vi "Modules - Communications V2.vi"() -> ()   [LabVIEW 2019]
uses:
  Controls/UDP - Event.ctl
  Controls/UDP - Status.ctl
  Controls/Communications - State.ctl
  Controls/eFGV States.ctl
  Controls/Communications - Data Structure.ctl
  Controls/FTDI - Communication.ctl
  Controls/UDP - Command.ctl
  Controls/Communication - Write Data.ctl
  Controls/UDP - Communication.ctl
  Controls/Global - Hold.vi
  Controls/Global - IP Address.vi
  Controls/Global - Handle.vi
  Controls/Global - Comport.vi
  Controls/Global - Device.vi
  Controls/Global - Data UDP.vi
  Controls/Global - Device Type.vi
  Controls/Global - Unit.vi
  Controls/Global - ADC.vi
  Controls/Global - PID.vi
  Controls/Global - System.vi
  Controls/Global - Test.vi
  Controls/Global - Channel.vi
  Controls/Global - Rendezvous.vi
  Controls/FGV States.ctl
panel:
  out "IP Registered":string[](array[string])
  out "Array":cluster{"error out":errorcluster, "IP":string}[](array[cluster])
  out "error out":errorcluster
  in  "timeout ms (25000)":i32=3000
  out "data out":string
  out "Array 2":T3(array[cluster]) {"Data"."Event" items=["Stop", "Running", "PID", "Up Limit", "Down Limit", "Load Limit"]; "Data"."Status" items=["Stop", "Ramp Up", "Ramp Down", "Jog Up", "Jog Down", "PID Mode", "PID Ramp"]}
  out "UDP Conn ref":refnum<k16>
  out "Stop":bool=TRUE
  out "IP":string[](array[string])
  out "Device":string[](array[string])
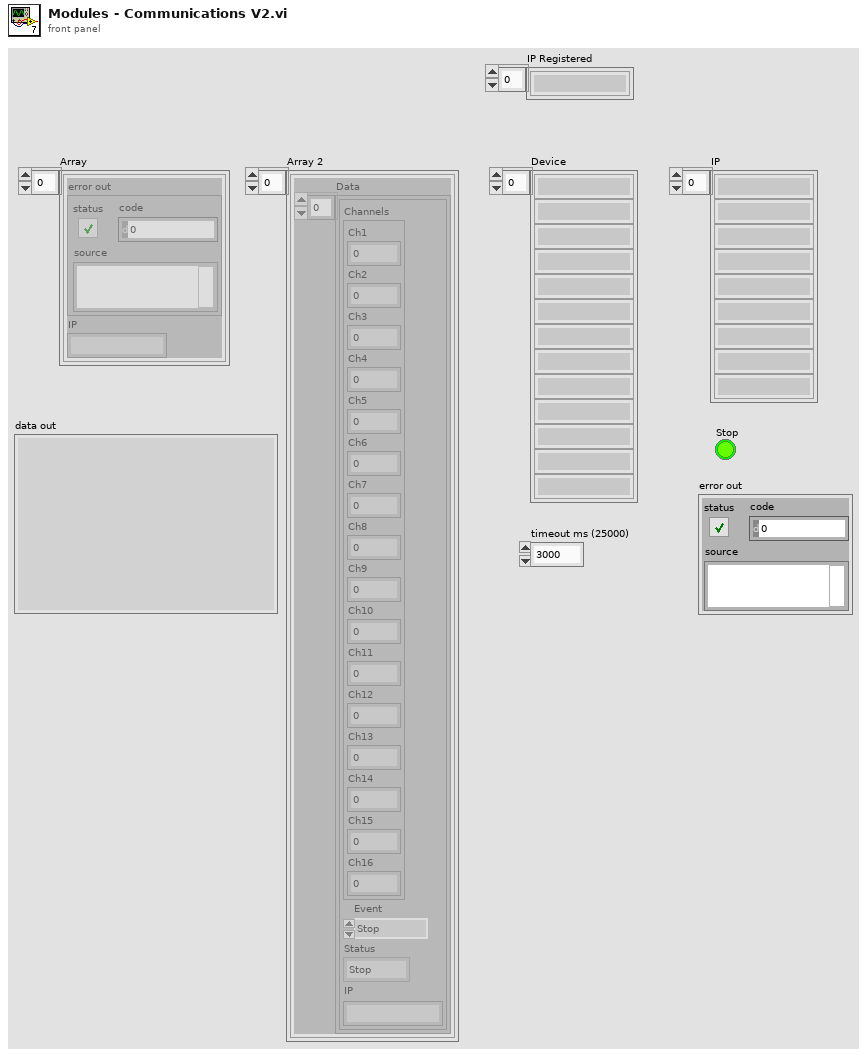
[diagram p1: front panel]
types:
  T1 = typedef "UDP - Event.ctl" = u16
  T2 = typedef "UDP - Status.ctl" = u16
  T3 = cluster{"Data":cluster{"Channels":cluster{"Ch1":sgl, "Ch2":sgl, "Ch3":sgl, "Ch4":sgl, "Ch5":sgl, "Ch6":sgl, "Ch7":sgl, "Ch8":sgl, "Ch9":sgl, "Ch10":sgl, "Ch11":sgl, "Ch12":sgl, "Ch13":sgl, "Ch14":sgl, "Ch15":sgl, "Ch16":sgl}, "Event":T1, "Status":T2, "IP":string}[]}[]
  T4 = cluster{"error out":errorcluster, "name":string}[]
  T5 = typedef "Communications - State.ctl" = enum16{"Init", "Idle", "Command", "Get IP Address", "Release Rendezvous", "Feedback", "Close"}
  T6 = enum32{"Invalid", "Standard", "Closed", "Hidden", "Minimized", "Maximized"}
  T7 = typedef "eFGV States.ctl" = enum16{"Init", "Read", "Write", "Exit"}
  T8 = typedef "Communications - Data Structure.ctl" = cluster{"UDP CMD":T9, "Unit?":bool, "Read Unit":bool[], "Trig?":bool, "UDP Info":cluster{"IP Address":string, "port":string, "UDP ref":refnum<k16>}[], "DataLogger":bool[], "VISA Ref":refnum<event-registration>, "Float":sgl, "Data":T11, "UDP Event Ref":refnum<event-registration>, "UDP ref":refnum<k16>, "Read Sensor":u8}
  T9 = typedef "FTDI - Communication.ctl" = cluster{"IP":string, "CMD":T10, "Port":string, "Datalog?":bool, "Float":dbl}
  T10 = typedef "UDP - Command.ctl" = enum16{"Stop", "Jog Up", "Jog Down", "Ramp Up", "Ramp Down", "PID Target", "PID Ramp", "Disp Run", "Read Ch Data", "Zero Channel", "Zero Disp", "Read Sensor", "Write Sensor", "Read ADC", "Write ADC", "Read PID", "Write PID", "Read Test", "Write Test", "Read System", "Write System", "Read Datalog", "Read Datalog Sensor"}
  T11 = typedef "Communication - Write Data.ctl" = cluster{"Test":cluster{"Target Load":sgl, "Target Disp":sgl, "Rate":sgl, "Speed":sgl}, "Sensor":cluster{"Name":string[], "Unit":string[], "Decimal Point":u8[], "Ch Log":u8[], "H Alarm":u8[], "L Alarm":u8[], "H Limit":sgl[], "L Limit":sgl[], "Filter":u8[], "Gain":u8[], "Calib Type":u32[]}, "PID":cluster{"SP":sgl, "PV":sgl, "kP":sgl, "kI":sgl, "kD":sgl, "FF":sgl, "Err Band":sgl, "Max":i32, "Min":i32, "Ts":u32, "Out":i32, "Mode":u8}, "ADC":cluster{"Active Ch":u8[], "Filter Type":u8, "Post Filter":u8[], "Gain":u8[], "FS":u16, "IntOC":u8, "IntFC":u8, "SysOC":u8, "Cofficient":dbl[], "K":dbl[], "Max":i32}, "System":cluster{"Out Type":u8, "Inverse":u8, "Monitor":u8, "Reserve":u8, "ACC Time":u32, "Pulse Rev":u32, "Stroke":u32, "Auto Off":u32, "Gear Ratio":sgl, "Pitch":sgl, "Max Speed":u32, "Jog Speed":u32, "Disp Coff":sgl, "Max Load":u32}, "Index":enum16{"Ch1", "Ch2", "Ch3", "Ch4", "Ch5", "Ch6", "Ch7", "Ch8", "Ch9", "Ch10", "Ch11", "Ch12", "Ch13", "Ch14", "Ch15", "Ch16"}, "Datalog":enum16{"Ch1-Ch16", "Ch17-Ch32", "Ch32-Ch48", "Ch49-Ch64", "Empty"}}
  T12 = cluster{"IP Address":string, "port":string, "UDP ref":refnum<k16>}
  T13 = enum16{"Ch1-Ch16", "Ch17-Ch32", "Ch32-Ch48", "Ch49-Ch64", "Empty"}
  T14 = cluster{"IP Address":string, "port":string, "UDP ref":refnum<k16>}[]
  T15 = typedef "FGV States.ctl" = enum16{"Read", "Write"}
  T16 = cluster{"Target Load":sgl, "Target Disp":sgl, "Rate":sgl, "Ch4":sgl}
  T17 = cluster{"Name":string[], "Unit":string[], "Decimal Point":u8[], "Ch Log":u8[], "H Alarm":u8[], "L Alarm":u8[], "H Limit":sgl[], "L Limit":sgl[], "Filter":u8[], "Gain":u8[], "Calib Type":u32[]}
  T18 = cluster{"SP":sgl, "PV":sgl, "kP":sgl, "kI":sgl, "kD":sgl, "FF":sgl, "Err Band":sgl, "Max":i32, "Min":i32, "Ts":u32, "Out":i32, "Mode":u8}
  T19 = cluster{"Active Ch":u8[], "Filter Type":u8, "Post Filter":u8[], "Gain":u8[], "FS":u16, "IntOC":u8, "IntFC":u8, "SysOC":u8, "Cofficient":dbl[], "K":dbl[], "Max":i32}
  T20 = cluster{"Out Type":u8, "Inverse":u8, "Monitor":u8, "Reserve":u8, "ACC Time":u32, "Pulse Rev":u32, "Stroke":u32, "Auto Off":u32, "Gear Ratio":sgl, "Pitch":sgl, "Max Speed":u32, "Jog Speed":u32, "Disp Coff":sgl, "Max Load":u32}
  T21 = cluster{"Name":string[], "Unit":string[], "Decimal Point":u8[], "Ch Log":u8[], "H Alarm":u8[], "L Alarm":u8[], "H Limit":sgl[], "L Limit":sgl[], "Filter":u8[], "Gain":u8[], "Calib Type":u32[]}[]
  T22 = cluster{"Active Ch":u8[], "Filter Type":u8, "Post Filter":u8[], "Gain":u8[], "FS":u16, "IntOC":u8, "IntFC":u8, "SysOC":u8, "Cofficient":dbl[], "K":dbl[], "Max":i32}[]
  T23 = cluster{"SP":sgl, "PV":sgl, "kP":sgl, "kI":sgl, "kD":sgl, "FF":sgl, "Err Band":sgl, "Max":i32, "Min":i32, "Ts":u32, "Out":i32, "Mode":u8}[]
  T24 = cluster{"Out Type":u8, "Inverse":u8, "Monitor":u8, "Reserve":u8, "ACC Time":u32, "Pulse Rev":u32, "Stroke":u32, "Auto Off":u32, "Gear Ratio":sgl, "Pitch":sgl, "Max Speed":u32, "Jog Speed":u32, "Disp Coff":sgl, "Max Load":u32}[]
  T25 = cluster{"Target Load":sgl, "Target Disp":sgl, "Rate":sgl, "Speed":sgl}
  T26 = cluster{"Target Load":sgl, "Target Disp":sgl, "Rate":sgl, "Speed":sgl}[]
  T27 = cluster{"Channels":cluster{"Ch1":sgl, "Ch2":sgl, "Ch3":sgl, "Ch4":sgl, "Ch5":sgl, "Ch6":sgl, "Ch7":sgl, "Ch8":sgl, "Ch9":sgl, "Ch10":sgl, "Ch11":sgl, "Ch12":sgl, "Ch13":sgl, "Ch14":sgl, "Ch15":sgl, "Ch16":sgl}, "Event":T1, "Status":T2, "IP":string}[]
  T28 = cluster{"Data":cluster{"Channels":cluster{"Ch1":sgl, "Ch2":sgl, "Ch3":sgl, "Ch4":sgl, "Ch5":sgl, "Ch6":sgl, "Ch7":sgl, "Ch8":sgl, "Ch9":sgl, "Ch10":sgl, "Ch11":sgl, "Ch12":sgl, "Ch13":sgl, "Ch14":sgl, "Ch15":sgl, "Ch16":sgl}, "Event":T1, "Status":T2, "IP":string}[]}
  T29 = typedef "Rendezvous RefNum" = refnum<k1>
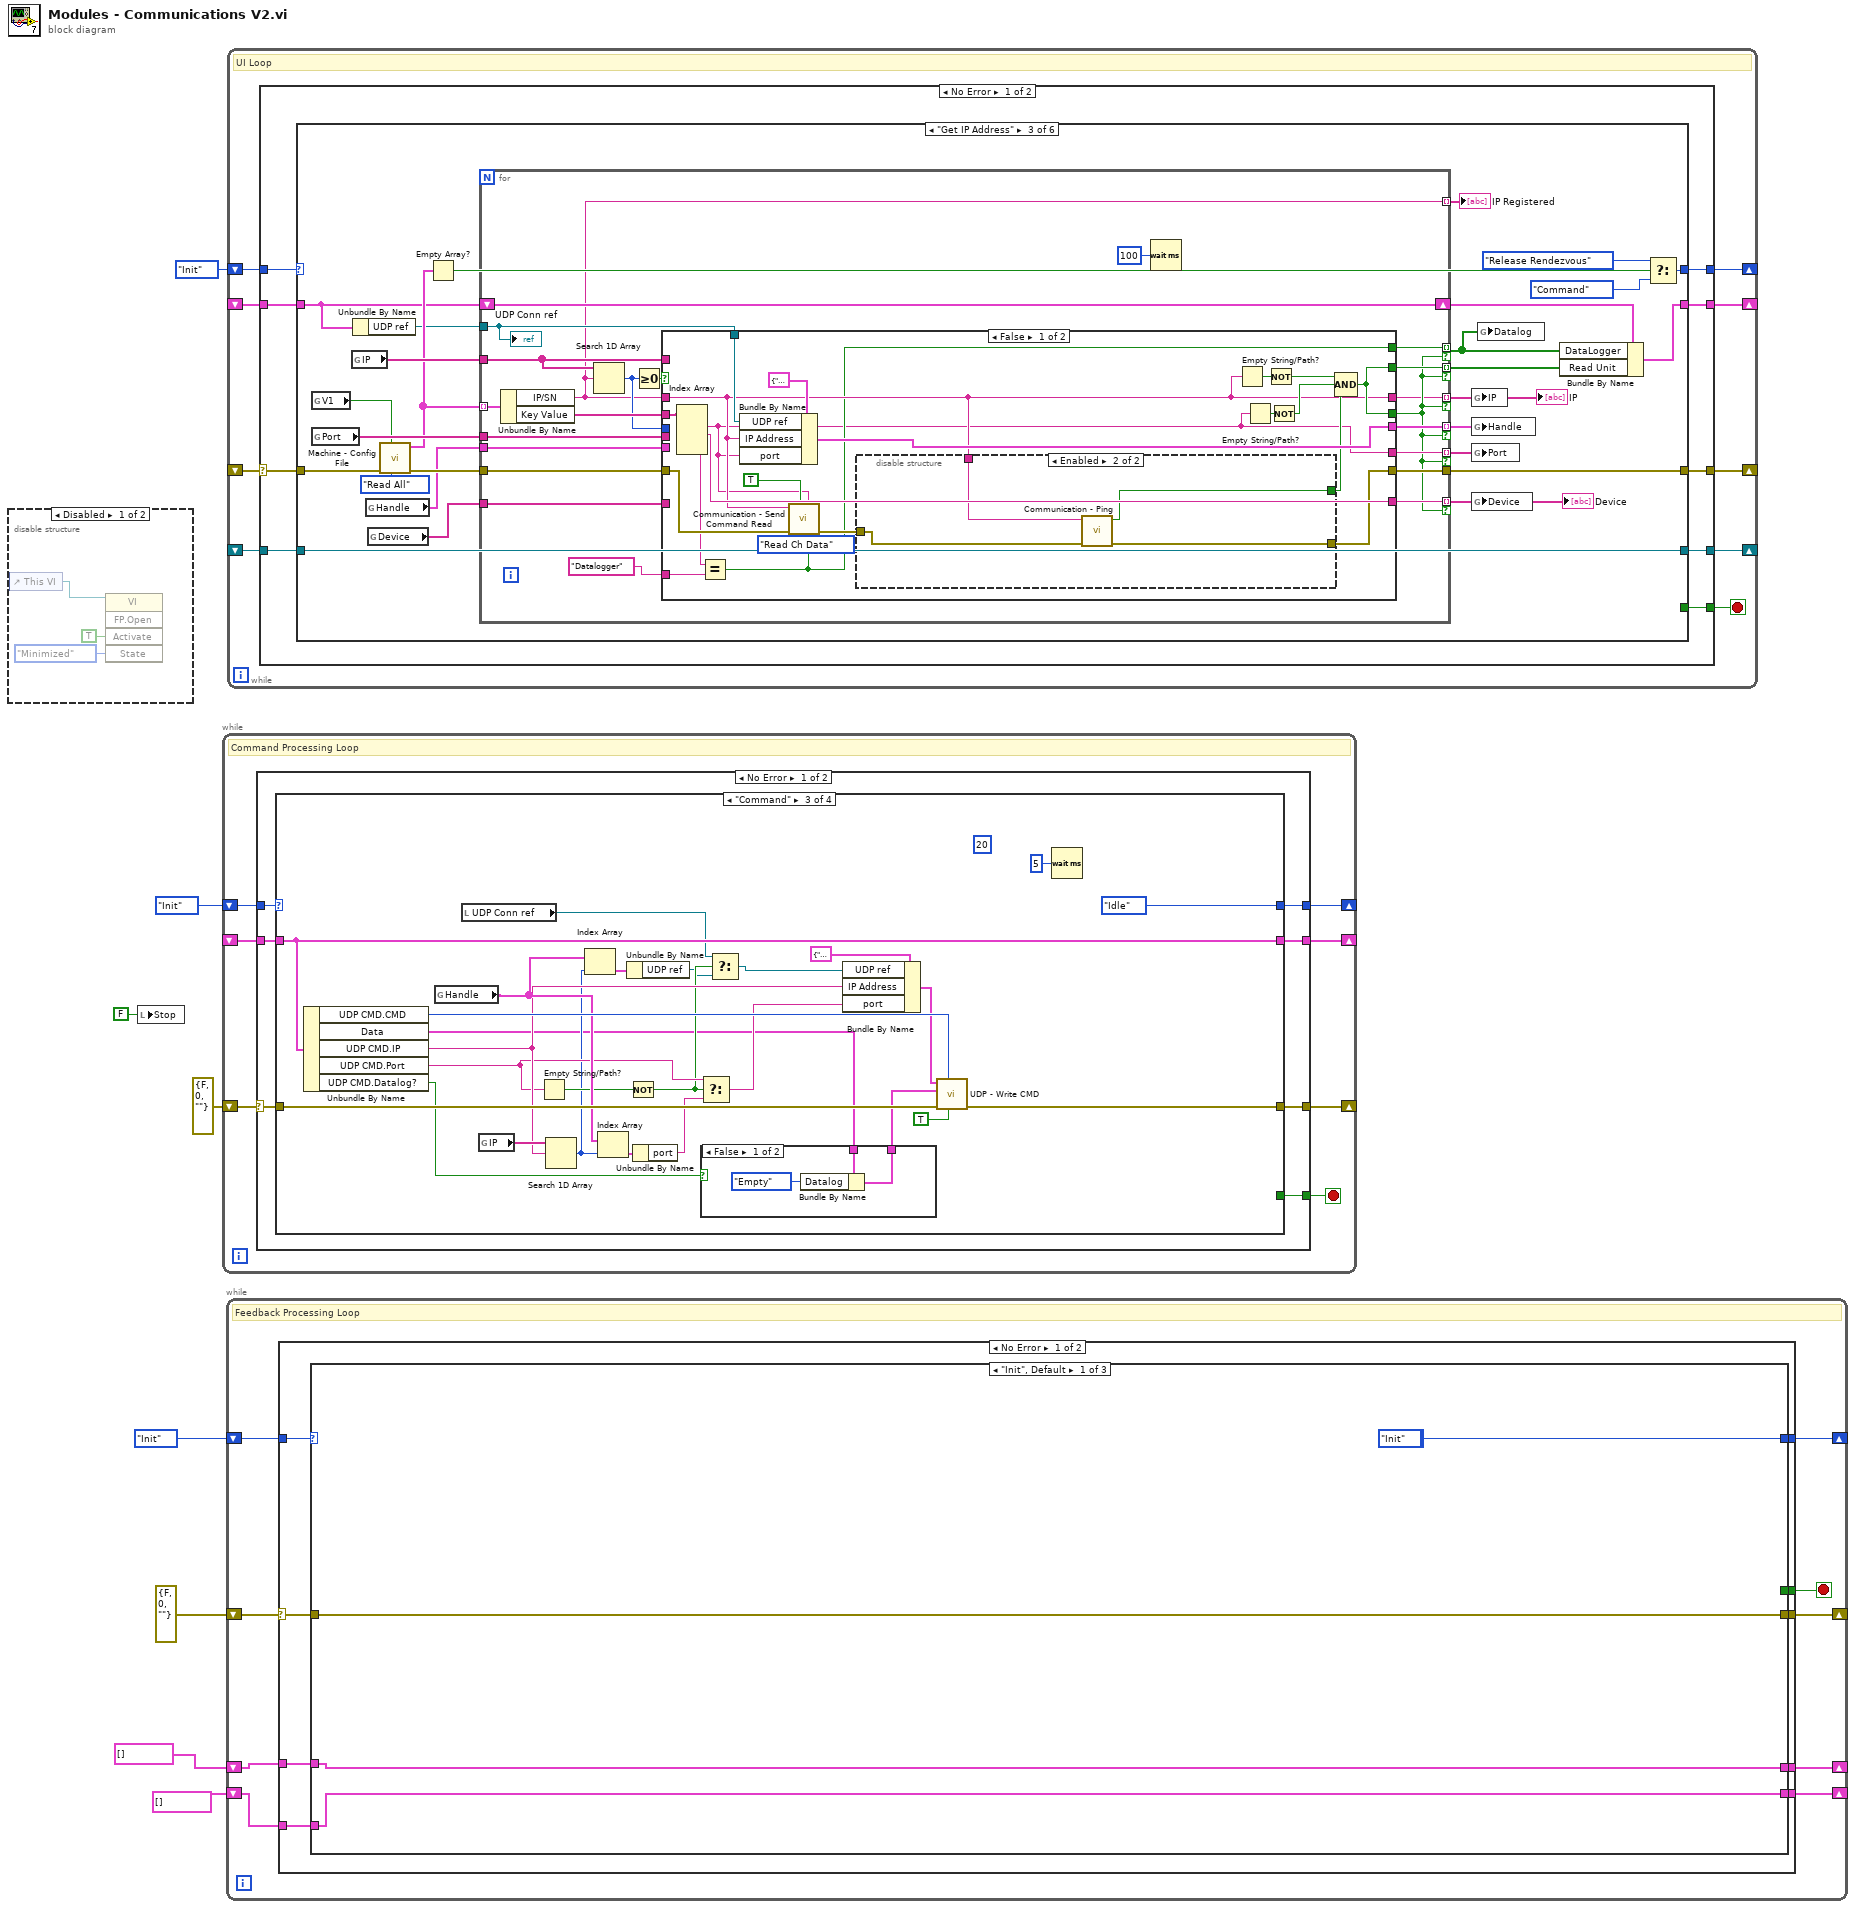
[diagram p0: block diagram]
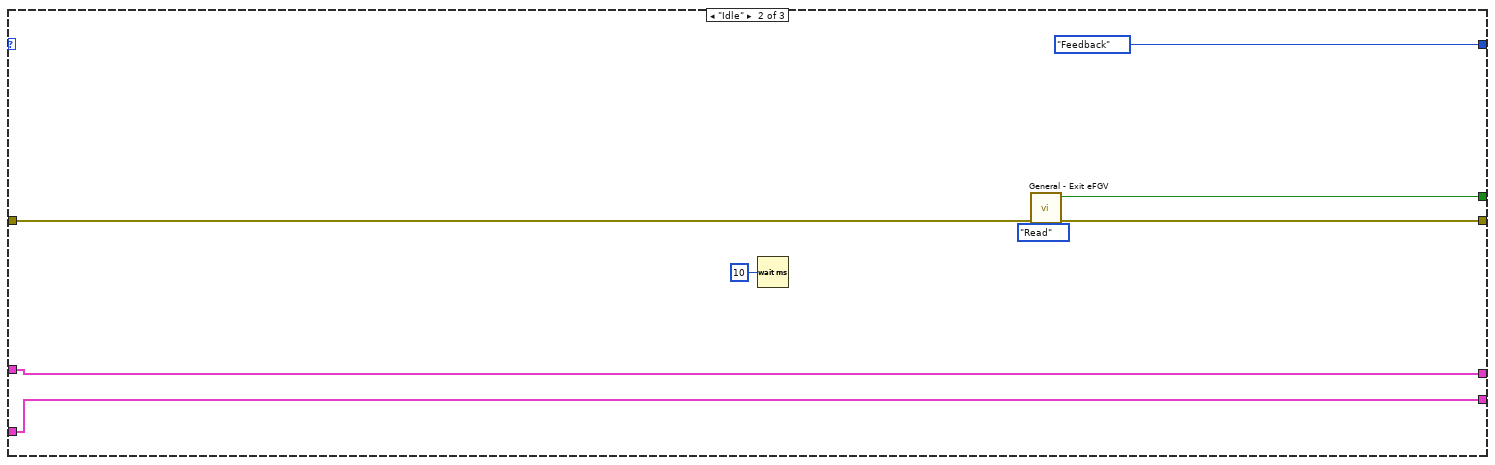
[diagram p3: hidden frame]
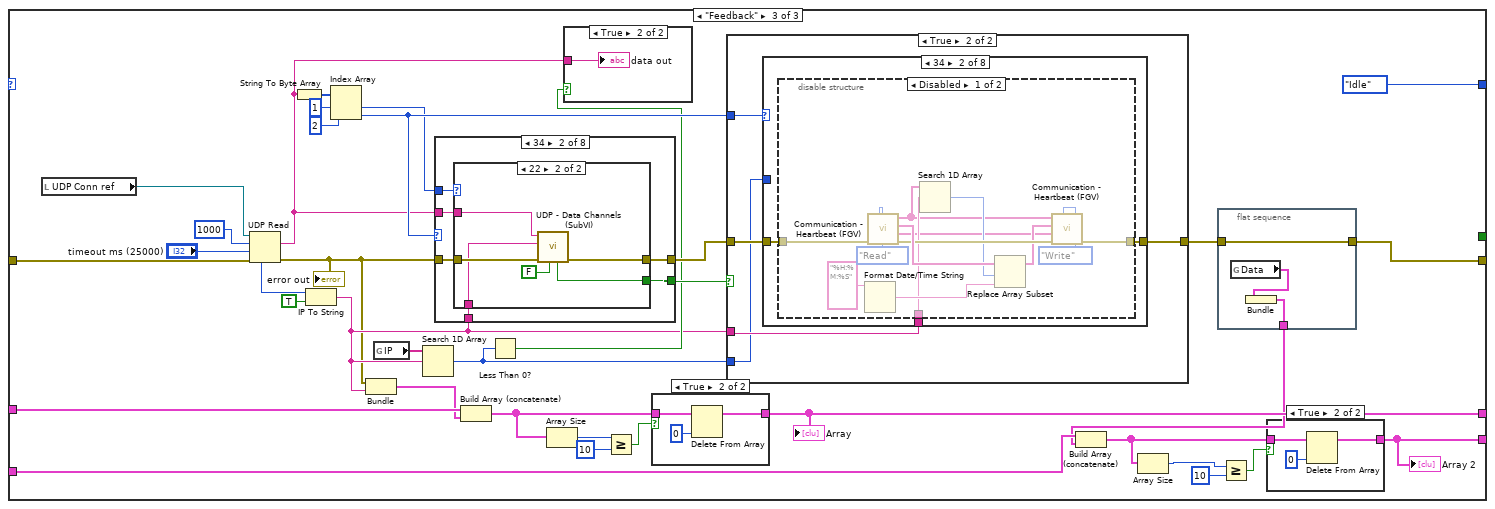
[diagram p4: hidden frame]
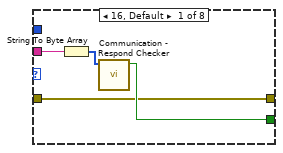
[diagram p8: hidden frame]
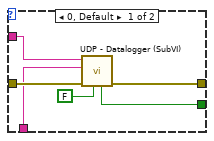
[diagram p9: hidden frame]
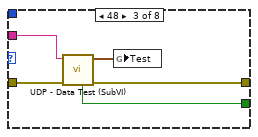
[diagram p10: hidden frame]
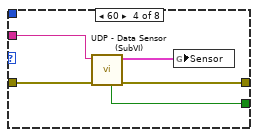
[diagram p11: hidden frame]
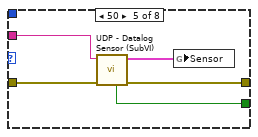
[diagram p12: hidden frame]
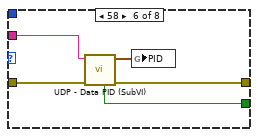
[diagram p13: hidden frame]
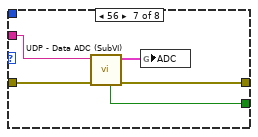
[diagram p14: hidden frame]
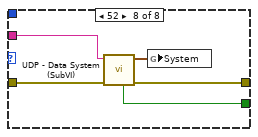
[diagram p15: hidden frame]
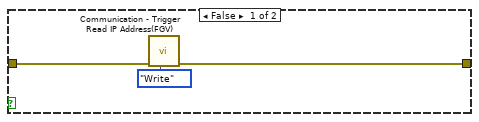
[diagram p16: hidden frame]
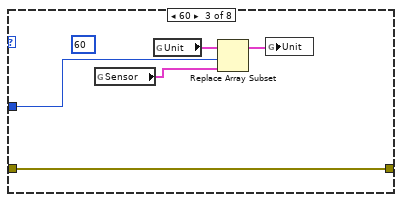
[diagram p19: hidden frame]
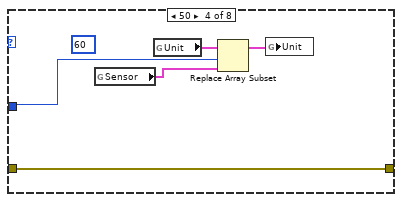
[diagram p20: hidden frame]
diagram:
  (unwired) Communications_-_State."Init"
  (unwired) Communications_-_State."Init"
  n1 = disable-structure shown="Disabled" {
    frame Disabled {
      n2 = control-ref of="This VI"() -> (w11:refnum<vi>)
      n3 = invoke class="VI" method="FP.Open"(reference=w11, "Activate"=TRUE ("Activate?"), "State"=T6."Minimized") -> ()  [unwired: 2 in, 5 out]
    }
    frame Enabled {
    }
  }
  n4 = local write "Stop"(FALSE ("Stop")) -> ()
  n5 = while {
    shift-right: [w17] -> _
    shift-left: errorcluster {"status"=FALSE, "code"=0, "source"=""} ("error IO") -> [w18]
    shift-right: [w15] -> _
    shift-left: Communications_-_State."Init" -> [w16]
    shift-right: [w13] -> _
    shift-left: _ -> [w12]
    stop <- w14 stop-if-true
    # "Command Processing Loop"
    n6 = case shown="No Error" w18 {
      selector: w18 -> [w24 w108]
      tunnel: [w25 w101] -> w17
      tunnel: w16 -> [w23 _]
      tunnel: [w22 Communications_-_State."Idle"] -> w15
      tunnel: [w21 _] -> w14
      tunnel: [w20 w110] -> w13
      tunnel: w12 -> [w19 w110]
      frame No Error {
        n7 = case shown="\"Command\"" w23 {
          tunnel: [w29 w43 w77 w98] -> w25
          tunnel: w24 -> [w27 w42 w87 w98]
          tunnel: [Communications_-_State."Idle" w37 Communications_-_State."Idle" Communications_-_State."Close"] -> w22
          tunnel: [_ _ _ TRUE] -> w21
          tunnel: [w31 w41 w86 w95] -> w20
          tunnel: w19 -> [_ w40 w86 w95]
          frame "Init", Default {
            n8 = call "Communication - UDP Command (eFGV).vi"("Action"=eFGV_States."Read", "error in"=w27) -> ("error out"=w30:errorcluster, "UDP Ref"=w28:refnum<user-event>)  [unwired: 7 in, 1 out]
            n9 = register-events(error in=w30, w28) -> (reference out=w26:refnum<event-registration>, error out=w29:errorcluster)  [unwired: 1 in]
            n10 = Bundle By Name(cluster=T8 {"UDP CMD"={"IP"="", "CMD"=enum."Stop", "Port"="", "Datalog?"=FALSE, "Float"=0.0}, "Unit?"=FALSE, "Read Unit"=[], "Trig?"=FALSE, "UDP Info"=[], "DataLogger"=[], "VISA Ref"=refnum, "Float"=0.0, "Data"={"Test"={"Target Load"=0.0, "Target Disp"=0.0, "Rate"=0.0, "Speed"=0.0}, "Sensor"={"Name"=[], "Unit"=[], "Decimal Point"=[], "Ch Log"=[], "H Alarm"=[], "L Alarm"=[], "H Limit"=[], "L Limit"=[], "Filter"=[], "Gain"=[], "Calib Type"=[]}, "PID"={"SP"=-2.7823365e-08, "PV"=-3.023652e-13, "kP"=8.5432666e-24, "kI"=2.29252e-41, "kD"=1.570387e-38, "FF"=25.0, "Err Band"=0.0, "Max"=15, "Min"=-7, "Ts"=1886611780, "Out"=0, "Mode"=0}, "ADC"={"Active Ch"=[255, 255, 255, 0, 0, 0, 0, 0], "Filter Type"=2, "Post Filter"=[1, 1, 1, 1, 0, 200, 66, 184], "Gain"=[0, 0, 0, 0, 0, 122, 68, 0], "FS"=32, "IntOC"=0, "IntFC"=255, "SysOC"=255, "Cofficient"=[1.0, 1.0, 1.0, 1.0, 1.0, 1.0, 1.0, 1.0], "K"=[1.2450000047683716, 1.2450000047683716], "Max"=1048576}, "System"={"Out Type"=0, "Inverse"=0, "Monitor"=0, "Reserve"=0, "ACC Time"=0, "Pulse Rev"=0, "Stroke"=0, "Auto Off"=0, "Gear Ratio"=0.0, "Pitch"=0.0, "Max Speed"=0, "Jog Speed"=0, "Disp Coff"=0.0, "Max Load"=0}, "Index"=enum."Ch1", "Datalog"=enum."Empty"}, "UDP Event Ref"=refnum, "UDP ref"=refnum, "Read Sensor"=0}, "UDP Event Ref"=w26) -> (w31:T8)
          }
          frame "Idle" {
            n11 = Unbundle By Name(w40) -> ("UDP Event Ref"=w44:refnum<event-registration>)
            n12 = event shown="[1] <UDP Ref>: User Event" {
              selector: w44 -> [_ _]
              dyn-events: _ -> [_ _]
              timeout: 1000 -> [_ _]
              tunnel: [w50 Communications_-_State."Command" ("f")] -> w38
              tunnel: [w47 w54] -> w43
              tunnel: w42 -> [w47 w54]
              tunnel: [w45 w62] -> w41
              tunnel: w40 -> [w45 w61]
              event Timeout {
                n13 = event-data() -> ()  [unwired: 1 in, 1 out]
                n14 = local read "Stop"() -> (w49:bool)
                n15 = Select(t=Communications_-_State."Close", s=w49, f=Communications_-_State."Idle") -> (s? t:f=w50:T5)
              }
              event User Event {
                n16 = event-data() -> ("IP"=w56:string, "CMD"=w60:T10, "Data"=w51:T11, "Port"=w53:string, "Datalog?"=w52:bool)  [unwired: 1 in]
                n17 = global read "Global - IP Address.vi" "IP"() -> (w59:string[])
                n18 = Index Array(array=w59, index=0) -> (element=w57:string)
                n19 = Equal?(x=w57, y=w56) -> ()  [unwired: 1 out]
                n20 = Bundle By Name(cluster=w61, "UDP CMD.IP"=w56, "UDP CMD.CMD"=w60, "Data"=w51, "UDP CMD.Port"=w53, "UDP CMD.Datalog?"=w52) -> (w62:T8)
              }
            }
            n21 = global read "Global - Hold.vi" "Hold"() -> (w39:bool)
            n22 = Select(t=Communications_-_State."Idle", s=w39, f=w38) -> (s? t:f=w37:T5)
          }
          frame "Command" {
            (unwired) 20
            n23 = Unbundle By Name(w86) -> ("UDP CMD.CMD"=w85:T10, "Data"=w65:T11, "UDP CMD.IP"=w79:string, "UDP CMD.Port"=w73:string, "UDP CMD.Datalog?"=w64:bool)
            n24 = global read "Global - Handle.vi" "Handle"() -> (w81:T14)
            n25 = local read "UDP Conn ref"() -> (w68:refnum<k16>)
            n26 = global read "Global - IP Address.vi" "IP"() -> (w83:string[])
            n27 = Empty String/Path?(string/path=w73) -> (empty?=w74:bool)
            n28 = Search 1D Array(1D array=w83, element=w79) -> (index of element=w67:i32)  [unwired: 1 in]
            n29 = Index Array(array=w81, index=w67) -> (element=w80:T12)
            n30 = Index Array(array=w81, index=w67) -> (element=w78:T12)
            n31 = Unbundle By Name(w80) -> ("UDP ref"=w69:refnum<k16>)
            n32 = Not(x=w74) -> (.not. x?=w70:bool)
            n33 = Unbundle By Name(w78) -> ("port"=w72:string)
            n34 = Select(t=w73, s=w70, f=w72) -> (s? t:f=w71:string)
            n35 = case shown="False" w64 {
              tunnel: w65 -> [w91 w94]
              tunnel: [w90 w93] -> w63
              frame False {
                n36 = Bundle By Name(cluster=w91, "Datalog"=T13."Empty") -> (w90:T11)
              }
              frame True {
                n37 = Bundle By Name(cluster=w94, "Datalog"=T13."Ch1-Ch16") -> (w93:T11)
              }
            }
            n38 = Select(t=w68, s=w70, f=w69) -> (s? t:f=w66:refnum<k16>)
            n39 = Bundle By Name(cluster=T12 {"IP Address"="", "port"="", "UDP ref"=refnum} ("element"), "UDP ref"=w66, "IP Address"=w79, "port"=w71) -> (w76:T12)
            n40 = call "UDP - Write CMD.vi"("V2"=TRUE, "CMD"=w85, "error in"=w87, "Data"=w63, "UDP Info"=w76) -> ("error out"=w77:errorcluster)  [unwired: 6 out]
            n41 = Wait (ms)(milliseconds to wait=u32 5) -> ()  [unwired: 1 out]
          }
          frame "Close" {
          }
        }
      }
      frame Error {
        n42 = global read "Global - IP Address.vi" "IP"() -> (w107:string[])
        n43 = Unbundle By Name(w108) -> ("source"=w103:string)
        n44 = Index Array(array=w107, index=0) -> (element=w105:string)
        n45 = Concatenate Strings(w105, " - " ("string"), w103) -> (w99:string)
        n46 = call <vilib>:"Clear Errors.vi"("error in (no error)"=w108) -> ("error out"=w102:errorcluster)  [unwired: 5 in, 1 out]
        n47 = call "General - Error Log eFGV.vi"("eFGV States"=eFGV_States."Write", "error in (no error)"=w102, "Error In"=w99) -> ("error out"=w101:errorcluster)  [unwired: 6 in, 2 out]
        n48 = Wait (ms)(milliseconds to wait=u32 100) -> ()  [unwired: 1 out]
      }
    }
  }
  n49 = while {
    shift-right: [w118] -> _
    shift-left: Communications_-_State."Init" -> [w119]
    shift-right: [w117] -> _
    shift-left: errorcluster {"status"=FALSE, "code"=0, "source"=""} ("error IO") -> [w120]
    shift-right: [w115] -> _
    shift-left: T4 [] -> [w114]
    shift-right: [w113] -> _
    shift-left: T3 [] -> [w112]
    stop <- w116 stop-if-true
    # "Feedback Processing Loop"
    n50 = case shown="No Error" w120 {
      selector: w120 -> [w126 w303]
      tunnel: w119 -> [w129 _]
      tunnel: [w128 Communications_-_State."Idle"] -> w118
      tunnel: [w127 w300] -> w117
      tunnel: [w125 _] -> w116
      tunnel: [w124 w299] -> w115
      tunnel: w114 -> [w123 w299]
      tunnel: [w122 w298] -> w113
      tunnel: w112 -> [w121 w298]
      frame No Error {
        n51 = case shown="\"Init\", Default" w129 {
          tunnel: [Communications_-_State."Idle" Communications_-_State."Feedback" Communications_-_State."Idle"] -> w128
          tunnel: [w132 w139 w150] -> w127
          tunnel: w126 -> [w132 w138 w165]
          tunnel: [_ w137 _] -> w125
          tunnel: [w131 w135 w158] -> w124
          tunnel: w123 -> [w131 w135 w162]
          tunnel: [w130 w134 w145] -> w122
          tunnel: w121 -> [w130 w134 w153]
          frame "Init", Default {
            (unwired) Communications_-_State."Init"
          }
          frame "Idle" {
            n52 = Wait (ms)(milliseconds to wait=u32 10) -> ()  [unwired: 1 out]
            n53 = call "General - Exit eFGV.vi"("eFGV States"=eFGV_States."Read", "error in (no error)"=w138) -> ("error out"=w139:errorcluster, "Exit Out"=w137:bool)  [unwired: 7 in, 1 out]
          }
          frame "Feedback" {
            n54 = local read "UDP Conn ref"() -> (w164:refnum<k16>)
            n55 = UDP Read(connection ID=w164, max size (548)=1000, timeout ms (25000)="timeout ms (25000)", 8:w165) -> (data out=w163:string, error out=w143:errorcluster, 6:w170:u32)  [unwired: 2 out]
            "error out" <- w143
            n56 = String To Byte Array(string=w163) -> (unsigned byte array=w174:u8[])
            n57 = IP To String(1:TRUE ("dot notation? (F)"), 2:w170) -> (0:w144:string)
            n58 = Index Array(array=w174, index #1=1 ("index"), index #2=2 ("index")) -> (element #1=w175:u8, element #2=w176:u8)
            n59 = Bundle("error out"=w143, "name"=w144) -> (w142:cluster{"error out":errorcluster, "name":string})  [unwired: 1 in]
            n60 = global read "Global - IP Address.vi" "IP"() -> (w173:string[])
            n61 = Search 1D Array(1D array=w173, element=w144) -> (index of element=w148:i32)  [unwired: 1 in]
            n62 = case shown="34" w176 {
              tunnel: [w191 w199 w216 w221 w226 w231 w236 w241] -> w172
              tunnel: [w192 w198 w215 w220 w225 w230 w235 w240] -> w171
              tunnel: w143 -> [w191 w195 w213 w218 w223 w228 w233 w238]
              tunnel: w163 -> [w190 w197 w212 w217 w222 w227 w232 w237]
              tunnel: w175 -> [_ w196 _ _ _ _ _ _]
              tunnel: w144 -> [_ w194 _ _ _ _ _ _]
              frame 16, Default {
                n63 = String To Byte Array(string=w190) -> (unsigned byte array=w193:u8[])
                n64 = call "Communication - Respond Checker.vi"("Read Data"=w193) -> ("Success"=w192:bool)  [unwired: 10 in]
              }
              frame 34 {
                n65 = case shown="22" w196 {
                  tunnel: [w203 w211] -> w199
                  tunnel: [w202 w210] -> w198
                  tunnel: w197 -> [w201 w208]
                  tunnel: w195 -> [w204 w207]
                  tunnel: w194 -> [w200 w206]
                  frame 0, Default {
                    n66 = call "UDP - Datalogger (SubVI).vi"("test?"=FALSE, "error in"=w204, "IP"=w200, "data in"=w201) -> ("error out"=w203:errorcluster, "Success"=w202:bool)  [unwired: 5 in, 1 out]
                  }
                  frame 22 {
                    n67 = call "UDP - Data Channels (SubVI).vi"("test?"=FALSE, "error in"=w207, "IP"=w206, "data in"=w208) -> ("error out"=w211:errorcluster, "Success"=w210:bool)  [unwired: 2 in, 4 out]
                  }
                }
              }
              frame 48 {
                n68 = call "UDP - Data Test (SubVI).vi"("error in"=w213, "data in"=w212) -> ("error out"=w216:errorcluster, "Data Test"=w214:T16, "Success"=w215:bool)  [unwired: 7 in]
                n69 = global write "Global - Data UDP.vi" "Test"(w214) -> ()
              }
              frame 60 {
                n70 = call "UDP - Data Sensor (SubVI).vi"("error in"=w218, "String"=w217) -> ("error out"=w221:errorcluster, "Sensor Out"=w219:T17, "Success"=w220:bool)  [unwired: 7 in]
                n71 = global write "Global - Data UDP.vi" "Sensor"(w219) -> ()
              }
              frame 50 {
                n72 = call "UDP - Datalog Sensor (SubVI).vi"("error in"=w223, "String"=w222) -> ("error out"=w226:errorcluster, "Sensor Out"=w224:T17, "Success"=w225:bool)  [unwired: 7 in]
                n73 = global write "Global - Data UDP.vi" "Sensor"(w224) -> ()
              }
              frame 58 {
                n74 = call "UDP - Data PID (SubVI).vi"("error in (no error)"=w228, "Data"=w227) -> ("error out"=w231:errorcluster, "PID Setting"=w229:T18, "Success"=w230:bool)  [unwired: 7 in]
                n75 = global write "Global - Data UDP.vi" "PID"(w229) -> ()
              }
              frame 56 {
                n76 = call "UDP - Data ADC (SubVI).vi"("error in (no error)"=w233, "Data"=w232) -> ("error out"=w236:errorcluster, "Data ADC"=w234:T19, "Success"=w235:bool)  [unwired: 7 in]
                n77 = global write "Global - Data UDP.vi" "ADC"(w234) -> ()
              }
              frame 52 {
                n78 = call "UDP - Data System (SubVI).vi"("error in (no error)"=w238, "Data"=w237) -> ("error out"=w241:errorcluster, "Data System"=w239:T20, "Success"=w240:bool)  [unwired: 7 in]
                n79 = global write "Global - Data UDP.vi" "System"(w239) -> ()
              }
            }
            n80 = Build Array (concatenate)(w162, w142) -> (w159:T4)
            n81 = Less Than 0?(x=w148) -> (x < 0?=w147:bool)
            n82 = Array Size(array=w159) -> (size(s)=w161:i32)
            n83 = case shown="True" w147 {
              tunnel: w163 -> [_ w178]
              frame False {
              }
              frame True {
                "data out" <- w178
              }
            }
            n84 = Greater Or Equal?(x=w161, y=10) -> (x >= y?=w157:bool)
            n85 = case shown="True" w157 {
              tunnel: w159 -> [w186 w189]
              tunnel: [w186 w188] -> w158
              frame False {
              }
              frame True {
                n86 = Delete From Array(array=w189, index=0) -> (array with subset deleted=w188:T4)  [unwired: 1 in, 1 out]
              }
            }
            "Array" <- w158
            n87 = case shown="True" w171 {
              tunnel: w172 -> [w242 w248]
              tunnel: [w243 w247] -> w149
              tunnel: w176 -> [_ w249]
              tunnel: w148 -> [_ w245]
              tunnel: w144 -> [_ w246]
              frame False {
                n88 = call "Communication - Trigger Read IP Address(FGV).vi"("Action"=eFGV_States."Write", "error in"=w242) -> ("error out"=w243:errorcluster)  [unwired: 7 in, 2 out]
              }
              frame True {
                n89 = case shown="34" w249 {
                  tunnel: w248 -> [w250 w253 w269 w274 w279 w287 w292 w297]
                  tunnel: [w250 w252 w269 w274 w279 w287 w292 w297] -> w247
                  tunnel: w245 -> [_ _ w268 w273 w278 w283 w288 w293]
                  tunnel: w246 -> [_ w251 _ _ _ _ _ _]
                  frame 0, Default {
                  }
                  frame 34 {
                    n90 = disable-structure shown="Disabled" {
                      disable-tunnel: w253 -> [w259 w267]
                      disable-tunnel: [w258 w267] -> w252
                      disable-tunnel: w251 -> [w257 _]
                      frame Disabled {
                        n91 = Format Date/Time String(time format string (%c)="%H:%M:%S") -> (date/time string=w263:string)  [unwired: 2 in]
                        n92 = call "Communication - Heartbeat (FGV).vi"("Action"=FGV_States."Read", "error in (no error)"=w259) -> ("error out"=w265:errorcluster, "Previous Out"=w254:string[], "Timestamp Out"=w266:string[], "IP Out"=w255:string[])  [unwired: 6 in]
                        n93 = Search 1D Array(1D array=w255, element=w257) -> (index of element=w256:i32)  [unwired: 1 in]
                        n94 = Replace Array Subset(array=w266, new element=w263, index=w256) -> (w264:string[])
                        n95 = call "Communication - Heartbeat (FGV).vi"("Action"=FGV_States."Write", "error in (no error)"=w265, "Previous"=w254, "Timestamp"=w264, "IP"=w255) -> ("error out"=w258:errorcluster)  [unwired: 3 in, 3 out]
                      }
                      frame Enabled {
                      }
                    }
                  }
                  frame 60 {
                    (unwired) u8 60 ("Numeric")
                    n96 = global read "Global - Data UDP.vi" "Sensor"() -> (w270:T17)
                    n97 = global read "Global - Unit.vi" "Unit"() -> (w271:T21)
                    n98 = Replace Array Subset(array=w271, new element=w270, index=w268) -> (w272:T21)
                    n99 = global write "Global - Unit.vi" "Unit"(w272) -> ()
                  }
                  frame 50 {
                    (unwired) u8 60 ("Numeric")
                    n100 = global read "Global - Data UDP.vi" "Sensor"() -> (w275:T17)
                    n101 = global read "Global - Unit.vi" "Unit"() -> (w276:T21)
                    n102 = Replace Array Subset(array=w276, new element=w275, index=w273) -> (w277:T21)
                    n103 = global write "Global - Unit.vi" "Unit"(w277) -> ()
                  }
                  frame 56 {
                    (unwired) u8 56 ("Numeric")
                    n104 = global read "Global - Data UDP.vi" "ADC"() -> (w280:T19)
                    n105 = global read "Global - ADC.vi" "ADC"() -> (w282:T22)
                    n106 = Replace Array Subset(array=w282, new element=w280, index=w278) -> (w281:T22)
                    n107 = global write "Global - ADC.vi" "ADC"(w281) -> ()
                  }
                  frame 58 {
                    (unwired) u8 58 ("Numeric")
                    n108 = global read "Global - Data UDP.vi" "PID"() -> (w284:T18)
                    n109 = global read "Global - PID.vi" "PID"() -> (w286:T23)
                    n110 = Replace Array Subset(array=w286, new element=w284, index=w283) -> (w285:T23)
                    n111 = global write "Global - PID.vi" "PID"(w285) -> ()
                  }
                  frame 52 {
                    (unwired) u8 52 ("Numeric")
                    n112 = global read "Global - Data UDP.vi" "System"() -> (w289:T20)
                    n113 = global read "Global - System.vi" "System"() -> (w291:T24)
                    n114 = Replace Array Subset(array=w291, new element=w289, index=w288) -> (w290:T24)
                    n115 = global write "Global - System.vi" "System"(w290) -> ()
                  }
                  frame 48 {
                    (unwired) u8 48 ("Numeric")
                    n116 = global read "Global - Data UDP.vi" "Test"() -> (w294:T25)
                    n117 = global read "Global - Test.vi" "Test"() -> (w295:T26)
                    n118 = Replace Array Subset(array=w295, new element=w294, index=w293) -> (w296:T26)
                    n119 = global write "Global - Test.vi" "Test"(w296) -> ()
                  }
                }
              }
            }
            n120 = Build Array (concatenate)(w153, w152) -> (w155:T3)
            n121 = Array Size(array=w155) -> (size(s)=w151:i32)
            n122 = flat-sequence {
              tunnel: [w181] -> w152
              tunnel: [w179] -> w150
              tunnel: w149 -> [w179]
              frame #0 {
                n123 = global read "Global - Channel.vi" "Data"() -> (w180:T27)
                n124 = Bundle("Data"=w180) -> (w181:T28)  [unwired: 1 in]
              }
            }
            n125 = Greater Or Equal?(x=w151, y=10) -> (x >= y?=w156:bool)
            n126 = case shown="True" w156 {
              tunnel: w155 -> [w182 w185]
              tunnel: [w182 w184] -> w145
              frame False {
              }
              frame True {
                n127 = Delete From Array(array=w185, index=0) -> (array with subset deleted=w184:T3)  [unwired: 1 in, 1 out]
              }
            }
            "Array 2" <- w145
          }
        }
      }
      frame Error {
        (unwired) Communications_-_State."Init"
        n128 = call <vilib>:"Clear Errors.vi"("error in (no error)"=w303) -> ("error out"=w300:errorcluster)  [unwired: 5 in, 1 out]
        n129 = Wait (ms)(milliseconds to wait=u32 100) -> ()  [unwired: 1 out]
      }
    }
  }
  n130 = while {
    shift-right: [w311] -> _
    shift-left: _ -> [w312]
    shift-right: [w309] -> _
    shift-left: Communications_-_State."Init" -> [w310]
    shift-right: [w308] -> _
    shift-left: _ -> [w307]
    shift-right: [w305] -> _
    shift-left: _ -> [w304]
    stop <- w306 stop-if-true
    # "UI Loop"
    n131 = case shown="No Error" w312 {
      selector: w312 -> [w320 w586]
      tunnel: [w321 w587] -> w311
      tunnel: w310 -> [w319 w581]
      tunnel: [w318 w581] -> w309
      tunnel: [w317 w592] -> w308
      tunnel: w307 -> [w316 w592]
      tunnel: [w315 _] -> w306
      tunnel: [w314 w591] -> w305
      tunnel: w304 -> [w313 w591]
      frame No Error {
        n132 = case shown="\"Get IP Address\"" w319 {
          tunnel: [w322 w354 w377 w525 w563 w572] -> w321
          tunnel: w320 -> [w335 w353 w388 w528 w562 w571]
          tunnel: [Communications_-_State."Get IP Address" w352 w374 w521 Communications_-_State."Idle" Communications_-_State."Close"] -> w318
          tunnel: [w337 w350 w391 w529 w565 w576] -> w317
          tunnel: w316 -> [_ w351 w391 w529 w565 w576]
          tunnel: [_ _ _ _ _ w574] -> w315
          tunnel: [w329 w349 w378 w520 w560 w573] -> w314
          tunnel: w313 -> [_ w348 w370 w520 w559 w573]
          frame "Init", Default {
            w334 = eFGV_States."Read" ("Action")
            n133 = call "Communication - Trigger Read IP Address(FGV).vi"("Action"=w334, "error in"=w335) -> ("error out"=w336:errorcluster, "Trigger ref"=w333:refnum<user-event>)  [unwired: 7 in, 1 out]
            n134 = call "General - Exit eFGV.vi"("eFGV States"=w334, "error in (no error)"=w336) -> ("error out"=w339:errorcluster, "Exit"=w338:refnum<user-event>)  [unwired: 7 in, 1 out]
            n135 = register-events(error in=w339, w338, w333) -> (reference out=w337:refnum<event-registration>, error out=w331:errorcluster)  [unwired: 1 in]
            n136 = global write "Global - IP Address.vi" "IP"(string[] [] ("IP")) -> ()
            n137 = global write "Global - Comport.vi" "Port"(string[] [] ("Port")) -> ()
            n138 = global write "Global - Device.vi" "Device"(string[] [] ("Device")) -> ()
            n139 = global write "Global - Handle.vi" "Handle"(T14 [] ("Handle")) -> ()
            n140 = global write "Global - Hold.vi" "Hold"(FALSE ("Hold")) -> ()
            n141 = call "UDP - Open Connection.vi"("CMD"=T8 {"UDP CMD"={"IP"="", "CMD"=enum."Stop", "Port"="", "Datalog?"=FALSE, "Float"=0.0}, "Unit?"=FALSE, "Read Unit"=[], "Trig?"=FALSE, "UDP Info"=[], "DataLogger"=[], "VISA Ref"=refnum, "Float"=0.0, "Data"={"Test"={"Target Load"=0.0, "Target Disp"=0.0, "Rate"=0.0, "Speed"=0.0}, "Sensor"={"Name"=[], "Unit"=[], "Decimal Point"=[], "Ch Log"=[], "H Alarm"=[], "L Alarm"=[], "H Limit"=[], "L Limit"=[], "Filter"=[], "Gain"=[], "Calib Type"=[]}, "PID"={"SP"=-2.7823365e-08, "PV"=-3.023652e-13, "kP"=8.5432666e-24, "kI"=2.29252e-41, "kD"=1.570387e-38, "FF"=25.0, "Err Band"=0.0, "Max"=15, "Min"=-7, "Ts"=1886611780, "Out"=0, "Mode"=0}, "ADC"={"Active Ch"=[255, 255, 255, 0, 0, 0, 0, 0], "Filter Type"=2, "Post Filter"=[1, 1, 1, 1, 0, 200, 66, 184], "Gain"=[0, 0, 0, 0, 0, 122, 68, 0], "FS"=32, "IntOC"=0, "IntFC"=255, "SysOC"=255, "Cofficient"=[1.0, 1.0, 1.0, 1.0, 1.0, 1.0, 1.0, 1.0], "K"=[1.2450000047683716, 1.2450000047683716], "Max"=1048576}, "System"={"Out Type"=0, "Inverse"=0, "Monitor"=0, "Reserve"=0, "ACC Time"=0, "Pulse Rev"=0, "Stroke"=0, "Auto Off"=0, "Gear Ratio"=0.0, "Pitch"=0.0, "Max Speed"=0, "Jog Speed"=0, "Disp Coff"=0.0, "Max Load"=0}, "Index"=enum."Ch1", "Datalog"=enum."Empty"}, "UDP Event Ref"=refnum, "UDP ref"=refnum, "Read Sensor"=0}, "error in"=w331, "UDP Info"=T12 {"IP Address"="192.168.88.100", "port"="4001", "UDP ref"=refnum}) -> ("error out"=w323:errorcluster, 5:w329:T8)  [unwired: 6 in, 1 out]
            n142 = disable-structure shown="Enabled" {
              disable-tunnel: w323 -> [w344 w346]
              disable-tunnel: [w343 w346] -> w322
              frame Enabled {
                n143 = call <vilib>:"System Exec.vi"("run minimized? (F)"=TRUE, "wait until completion? (T)"=FALSE, "error in (no error)"=w344, "command line"="\"C:\\laragon\\bin\\python\\python-3.10\\python.exe\" \"C:\\laragon\\www\\ping.py\"") -> ("error out"=w343:errorcluster)  [unwired: 4 in, 3 out]
              }
              frame Disabled {
              }
            }
          }
          frame "Idle" {
            n144 = event shown="[0] Timeout" {
              selector: w351 -> [_ _ _]
              dyn-events: [_ _ _] -> w350
              timeout: 1000 -> [_ _ _]
              tunnel: [w357 w362 w365] -> w354
              tunnel: w353 -> [w357 w362 w365]
              tunnel: [Communications_-_State."Get IP Address" Communications_-_State."Get IP Address" Communications_-_State."Close"] -> w352
              tunnel: [w355 w360 w363] -> w349
              tunnel: w348 -> [w355 w359 w363]
              event Timeout {
                n145 = event-data() -> ()  [unwired: 1 in, 3 out]
              }
              event User Event {
                n146 = event-data() -> ()  [unwired: 1 in, 1 out]
                n147 = Bundle By Name(cluster=w359, "Trig?"=TRUE) -> (w360:T8)
              }
              event User Event {
                n148 = event-data() -> ()  [unwired: 1 in, 5 out]
              }
            }
          }
          frame "Get IP Address" {
            n149 = global read "Global - Data UDP.vi" "V1"() -> (w367:bool)
            n150 = global read "Global - Comport.vi" "Port"() -> (w380:string[])
            n151 = global read "Global - IP Address.vi" "IP"() -> (w384:string[])
            n152 = Unbundle By Name(w370) -> ("UDP ref"=w369:refnum<k16>)
            n153 = global read "Global - Handle.vi" "Handle"() -> (w383:T14)
            n154 = global read "Global - Device.vi" "Device"() -> (w382:string[])
            n155 = call "Machine - Config File.vi"("Action"=enum16{"Write", "Read", "Read All", "Remove"}."Read All", "V1"=w367, "error in (no error)"=w388) -> ("error out"=w389:errorcluster, "Value Out"=w376:cluster{"IP/SN":string, "Key Value":string[]}[])  [unwired: 7 in]
            n156 = Empty Array?(array=w376) -> (empty?=w373:bool)
            n157 = for {
              tunnel: w389 -> [w412]
              tunnel: [w413] -> w377
              tunnel: [w394] -> w387 mode=indexing if=w395
              tunnel: [w400] -> w386 mode=indexing if=w395
              tunnel: w376 -> [w411] mode=indexing
              tunnel: [w409] -> w385 mode=indexing if=w395
              tunnel: w384 -> [w407]
              tunnel: w383 -> [w402]
              tunnel: w382 -> [w406]
              tunnel: [w405] -> w381 mode=indexing if=w395
              tunnel: w380 -> [w404]
              tunnel: [w403] -> w379 mode=indexing if=w395
              shift-right: [w399] -> w371
              shift-left: w370 -> [w399]
              tunnel: w369 -> [w397]
              tunnel: [w396] -> w368 mode=indexing if=w395
              tunnel: [w393] -> w366 mode=indexing
              n158 = Unbundle By Name(w411) -> ("IP/SN"=w393:string, "Key Value"=w410:string[])
              n159 = Search 1D Array(1D array=w407, element=w393) -> (index of element=w401:i32)  [unwired: 1 in]
              n160 = Greater Or Equal To 0?(x=w401) -> (x >= 0?=w408:bool)
              n161 = case shown="False" w408 {
                tunnel: [w420 w479] -> w413
                tunnel: w412 -> [w422 w467]
                tunnel: w410 -> [w433 w477]
                tunnel: [w432 w483] -> w409
                tunnel: [w425 w480] -> w400
                tunnel: [w428 w478] -> w395
                tunnel: w393 -> [w418 _]
                tunnel: [w418 w472] -> w394
                tunnel: w407 -> [_ w486]
                tunnel: w401 -> [_ w482]
                tunnel: w402 -> [_ w485]
                tunnel: w406 -> [_ w484]
                tunnel: [w414 w471] -> w405
                tunnel: w404 -> [_ w481]
                tunnel: [w428 w478] -> w403
                tunnel: w397 -> [w426 _]
                tunnel: "Datalogger" -> [w417 w474]
                tunnel: [w415 w473] -> w396
                frame False {
                  n162 = Index Array(array=w433) -> (element #1=w414:string, element #2=w432:string, element #4=w416:string)  [unwired: 4 in, 1 out]
                  n163 = Equal?(x=w416, y=w417) -> (x = y?=w415:bool)
                  n164 = Bundle By Name(cluster=T12 {"IP Address"="192.168.88.49", "port"="", "UDP ref"=refnum} ("UDP Info"), "UDP ref"=w426, "IP Address"=w418, "port"=w414) -> (w425:T12)
                  n165 = call "Communication - Send Command Read.vi"("Datalog?"=w415, "Port"=w414, "Bypass?"=TRUE, "error in (no error)"=w422, "Action"=UDP_-_Command."Read Ch Data", "Device IP Address"=w418) -> ("error out"=w421:errorcluster)  [unwired: 5 in]
                  n166 = disable-structure shown="Enabled" {
                    disable-tunnel: w421 -> [w438 w465]
                    disable-tunnel: [w437 w466] -> w420
                    disable-tunnel: [w436 w463] -> w419
                    disable-tunnel: w418 -> [w435 w464]
                    frame Disabled {
                      n167 = for {
                        N: 20 -> [_]
                        tunnel: w435 -> [w450]
                        tunnel: [w445] -> w436
                        shift-right: [w446] -> w437
                        shift-left: w438 -> [w451]
                        stop <- w445 stop-if-true
                        n168 = Wait (ms)(milliseconds to wait=u32 100) -> ()  [unwired: 1 out]
                        n169 = call "Communication - Heartbeat (FGV).vi"("Action"=FGV_States."Read", "error in (no error)"=w451) -> ("error out"=w447:errorcluster, "Previous Out"=w444:string[], "Timestamp Out"=w440:string[], "IP Out"=w441:string[])  [unwired: 6 in]
                        n170 = Search 1D Array(1D array=w441, element=w450) -> (index of element=w442:i32)  [unwired: 1 in]
                        n171 = Index Array(array=w440, index=w442) -> (element=w443:string)
                        n172 = Index Array(array=w444, index=w442) -> (element=w449:string)
                        n173 = Not Equal?(x=w443, y=w449) -> (x != y?=w445:bool)
                        n174 = case shown="True" w445 {
                          tunnel: w447 -> [w453 w461]
                          tunnel: [w453 w460] -> w446
                          tunnel: w444 -> [_ w459]
                          tunnel: w443 -> [_ w458]
                          tunnel: w442 -> [_ w457]
                          tunnel: w441 -> [_ w455]
                          tunnel: w440 -> [_ w454]
                          frame False {
                          }
                          frame True {
                            n175 = Replace Array Subset(array=w459, new element=w458, index=w457) -> (w456:string[])
                            n176 = call "Communication - Heartbeat (FGV).vi"("Action"=FGV_States."Write", "error in (no error)"=w461, "Previous"=w456, "Timestamp"=w454, "IP"=w455) -> ("error out"=w460:errorcluster)  [unwired: 3 in, 3 out]
                          }
                        }
                      }
                    }
                    frame Enabled {
                      n177 = call "Communication - Ping.vi"("error in"=w465, "IP"=w464) -> ("error out"=w466:errorcluster, "Active?"=w463:bool)  [unwired: 7 in, 1 out]
                    }
                  }
                  n178 = Empty String/Path?(string/path=w418) -> (empty?=w434:bool)
                  n179 = Empty String/Path?(string/path=w414) -> (empty?=w431:bool)
                  n180 = Not(x=w434) -> (.not. x?=w430:bool)
                  n181 = Not(x=w431) -> (.not. x?=w429:bool)
                  n182 = Compound Arithmetic op=AND(w430, w429, w419) -> (w428:bool)
                }
                frame True {
                  n183 = Index Array(array=w484, index=w482) -> (element=w483:string)
                  n184 = Index Array(array=w477, index=3) -> (element=w475:string)
                  n185 = Index Array(array=w486, index=w482) -> (element=w472:string)
                  n186 = Index Array(array=w485, index=w482) -> (element=w480:T12)
                  n187 = Index Array(array=w481, index=w482) -> (element=w471:string)
                  n188 = Equal?(x=w475, y=w474) -> (x = y?=w473:bool)
                  n189 = call "Communication - Send Command Read.vi"("Datalog?"=w473, "Port"=w471, "Bypass?"=TRUE, "error in (no error)"=w467, "Action"=UDP_-_Command."Read Ch Data", "Device IP Address"=w472) -> ("error out"=w468:errorcluster)  [unwired: 5 in]
                  n190 = disable-structure shown="Enabled" {
                    disable-tunnel: [w490 w517] -> w479
                    disable-tunnel: w468 -> [w489 w516]
                    disable-tunnel: w472 -> [w488 w518]
                    disable-tunnel: [w487 w515] -> w478
                    frame Disabled {
                      n191 = for {
                        N: 20 -> [_]
                        tunnel: w488 -> [w502]
                        tunnel: [w497] -> w487
                        shift-right: [w498] -> w490
                        shift-left: w489 -> [w503]
                        stop <- w497 stop-if-true
                        n192 = Wait (ms)(milliseconds to wait=u32 100) -> ()  [unwired: 1 out]
                        n193 = call "Communication - Heartbeat (FGV).vi"("Action"=FGV_States."Read", "error in (no error)"=w503) -> ("error out"=w499:errorcluster, "Previous Out"=w496:string[], "Timestamp Out"=w492:string[], "IP Out"=w493:string[])  [unwired: 6 in]
                        n194 = Search 1D Array(1D array=w493, element=w502) -> (index of element=w494:i32)  [unwired: 1 in]
                        n195 = Index Array(array=w492, index=w494) -> (element=w495:string)
                        n196 = Index Array(array=w496, index=w494) -> (element=w501:string)
                        n197 = Not Equal?(x=w495, y=w501) -> (x != y?=w497:bool)
                        n198 = case shown="True" w497 {
                          tunnel: w499 -> [w505 w513]
                          tunnel: [w505 w512] -> w498
                          tunnel: w496 -> [_ w511]
                          tunnel: w495 -> [_ w510]
                          tunnel: w494 -> [_ w509]
                          tunnel: w493 -> [_ w507]
                          tunnel: w492 -> [_ w506]
                          frame False {
                          }
                          frame True {
                            n199 = Replace Array Subset(array=w511, new element=w510, index=w509) -> (w508:string[])
                            n200 = call "Communication - Heartbeat (FGV).vi"("Action"=FGV_States."Write", "error in (no error)"=w513, "Previous"=w508, "Timestamp"=w506, "IP"=w507) -> ("error out"=w512:errorcluster)  [unwired: 3 in, 3 out]
                          }
                        }
                      }
                    }
                    frame Enabled {
                      n201 = call "Communication - Ping.vi"("error in"=w516, "IP"=w518) -> ("error out"=w517:errorcluster, "Active?"=w515:bool)  [unwired: 7 in, 1 out]
                    }
                  }
                }
              }
              n202 = Wait (ms)(milliseconds to wait=u32 100) -> ()  [unwired: 1 out]
              "UDP Conn ref" <- w397
            }
            "IP" <- w387
            "Device" <- w385
            "IP Registered" <- w366
            n203 = global write "Global - IP Address.vi" "IP"(w387) -> ()
            n204 = global write "Global - Handle.vi" "Handle"(w386) -> ()
            n205 = global write "Global - Comport.vi" "Port"(w381) -> ()
            n206 = global write "Global - Device.vi" "Device"(w385) -> ()
            n207 = global write "Global - Device Type.vi" "Datalog"(w368) -> ()
            n208 = Bundle By Name(cluster=w371, "DataLogger"=w368, "Read Unit"=w379) -> (w378:T8)
            n209 = Select(t=Communications_-_State."Release Rendezvous", s=w373, f=Communications_-_State."Command") -> (s? t:f=w374:T5)
          }
          frame "Command" {
            n210 = Unbundle By Name(w520) -> ("Trig?"=w524:bool, "Read Unit"=w526:bool[], "DataLogger"=w519:bool[])
            n211 = global read "Global - Handle.vi" "Handle"() -> (w527:T14)
            n212 = for {
              shift-right: [w533] -> w525
              shift-left: w528 -> [w534]
              tunnel: w527 -> [w532] mode=indexing
              tunnel: w526 -> [w531] mode=indexing
              tunnel: w519 -> [w530] mode=indexing
              n213 = case shown="True" w531 {
                tunnel: w534 -> [w535 w539]
                tunnel: [w535 w538] -> w533
                tunnel: w532 -> [_ w537]
                tunnel: w530 -> [_ w536]
                frame False {
                }
                frame True {
                  n214 = case shown="True" w536 {
                    tunnel: w539 -> [w545 w549]
                    tunnel: [w544 w548] -> w538
                    tunnel: w537 -> [w542 w547]
                    frame False {
                      n215 = call "UDP - Write CMD.vi"("V2"=TRUE, "CMD"=UDP_-_Command."Read Sensor", "error in"=w545, "UDP Info"=w542) -> ("error out"=w544:errorcluster)  [unwired: 1 in, 6 out]
                      n216 = Wait (ms)(milliseconds to wait=u32 10) -> ()  [unwired: 1 out]
                    }
                    frame True {
                      n217 = for {
                        N: 16 -> [_]
                        tunnel: w547 -> [w555]
                        shift-right: [w557] -> w548
                        shift-left: w549 -> [w558]
                        i -> [w552]
                        n218 = Bundle By Name(cluster=T11 {"Test"={"Target Load"=0.0, "Target Disp"=0.0, "Rate"=0.0, "Speed"=0.0}, "Sensor"={"Name"=[], "Unit"=[], "Decimal Point"=[], "Ch Log"=[], "H Alarm"=[], "L Alarm"=[], "H Limit"=[], "L Limit"=[], "Filter"=[], "Gain"=[], "Calib Type"=[]}, "PID"={"SP"=-2.7823365e-08, "PV"=-3.023652e-13, "kP"=8.5432666e-24, "kI"=2.29252e-41, "kD"=1.570387e-38, "FF"=25.0, "Err Band"=0.0, "Max"=15, "Min"=-7, "Ts"=1886611780, "Out"=0, "Mode"=0}, "ADC"={"Active Ch"=[255, 255, 255, 0, 0, 0, 0, 0], "Filter Type"=2, "Post Filter"=[1, 1, 1, 1, 0, 200, 66, 184], "Gain"=[0, 0, 0, 0, 0, 122, 68, 0], "FS"=32, "IntOC"=0, "IntFC"=255, "SysOC"=255, "Cofficient"=[1.0, 1.0, 1.0, 1.0, 1.0, 1.0, 1.0, 1.0], "K"=[1.2450000047683716, 1.2450000047683716], "Max"=1048576}, "System"={"Out Type"=0, "Inverse"=0, "Monitor"=0, "Reserve"=0, "ACC Time"=0, "Pulse Rev"=0, "Stroke"=0, "Auto Off"=0, "Gear Ratio"=0.0, "Pitch"=0.0, "Max Speed"=0, "Jog Speed"=0, "Disp Coff"=0.0, "Max Load"=0}, "Index"=enum."Ch1", "Datalog"=enum."Empty"} ("Data"), "Index"=w552) -> (w551:T11)
                        n219 = call "UDP - Write CMD.vi"("V2"=TRUE, "CMD"=UDP_-_Command."Read Datalog Sensor", "error in"=w558, "Data"=w551, "UDP Info"=w555) -> ("error out"=w557:errorcluster)  [unwired: 6 out]
                        n220 = Wait (ms)(milliseconds to wait=u32 10) -> ()  [unwired: 1 out]
                      }
                    }
                  }
                }
              }
            }
            n221 = Select(t=Communications_-_State."Idle", s=w524, f=Communications_-_State."Release Rendezvous") -> (s? t:f=w521:T5)
          }
          frame "Release Rendezvous" {
            n222 = disable-structure shown="Enabled" {
              disable-tunnel: [w568 w569] -> w563
              disable-tunnel: w562 -> [w567 w569]
              frame Disabled {
                n223 = global read "Global - Rendezvous.vi" "rendezvous"() -> (w566:T29)
                n224 = call <vilib>:"Wait at Rendezvous.vi"("error in (no error)"=w567, "rendezvous"=w566) -> ("error out"=w568:errorcluster)  [unwired: 3 in, 2 out]
              }
              frame Enabled {
              }
            }
            n225 = Bundle By Name(cluster=w559, "Trig?"=TRUE) -> (w560:T8)
          }
          frame "Close" {
            w574 = TRUE
            n226 = global read "Global - Handle.vi" "Handle"() -> (w570:T14)
            n227 = for {
              tunnel: w570 -> [w580] mode=indexing
              shift-right: [w578] -> w572
              shift-left: w571 -> [w579]
              n228 = Unbundle By Name(w580) -> ("UDP ref"=w577:refnum<k16>)
              n229 = UDP Close(connection ID=w577, 8:w579) -> (error out=w578:errorcluster)  [unwired: 1 out]
            }
            "Stop" <- w574
          }
        }
      }
      frame Error {
        n230 = Unbundle By Name(w586) -> ("source"=w584:string)
        n231 = Concatenate Strings("UI Loop (Comm)" ("string"), " - " ("string"), w584) -> (w582:string)
        n232 = Wait (ms)(milliseconds to wait=u32 100) -> ()  [unwired: 1 out]
        n233 = call <vilib>:"Clear Errors.vi"("error in (no error)"=w586) -> ("error out"=w588:errorcluster)  [unwired: 5 in, 1 out]
        n234 = call "General - Error Log eFGV.vi"("eFGV States"=eFGV_States."Write", "error in (no error)"=w588, "Error In"=w582) -> ("error out"=w587:errorcluster)  [unwired: 6 in, 2 out]
      }
    }
  }
